vi "sort files in folder by integer in filename.vi"(11 "subarray":string[](array[string])) -> (3 "elements":string[](array[string]))   [LabVIEW 2020]
uses:
  <userlib>/_OpenG.lib/array/array.llb/Sort 1D Array (I32)__ogtk.vi
  <userlib>/_OpenG.lib/array/array.llb/Index 1D Array Elements (String)__ogtk.vi
panel:
  out "number":i32
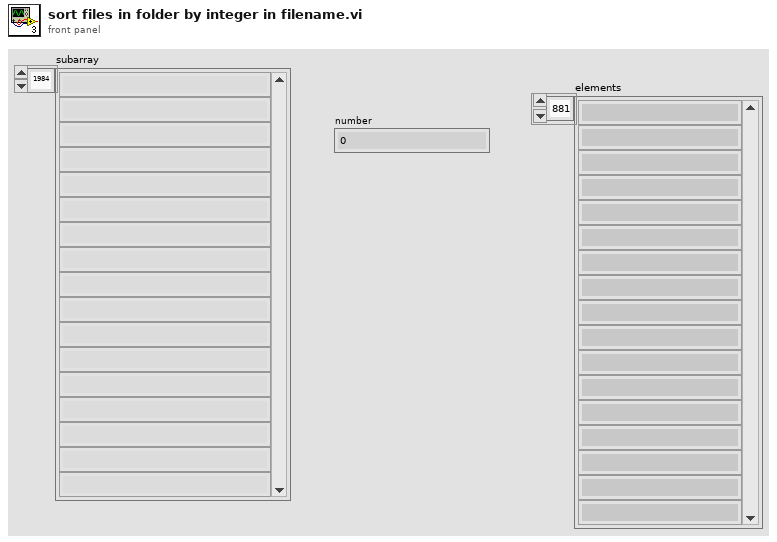
[diagram p1: front panel]
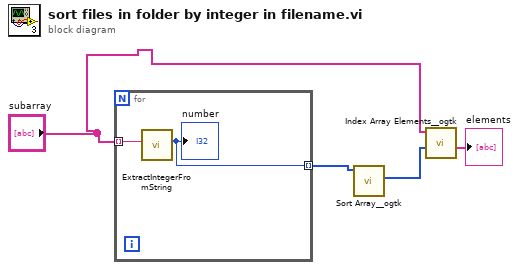
[diagram p0: block diagram]
diagram:
  n1 = for {
    tunnel: "subarray" -> [w6] mode=indexing
    tunnel: [w5] -> w4 mode=indexing
    n2 = call "ExtractIntegerFromString.vi"("String"=w6) -> ("number"=w5:i32)  [unwired: 10 in]
    "number" <- w5
  }
  n3 = call-poly <userlib>:"Sort Array__ogtk.vi"("Array in"=w4) -> ("Sorted Pointers"=w2:i32[])  [unwired: 9 in, 1 out]
  n4 = call-poly <userlib>:"Index Array Elements__ogtk.vi"("indices"=w2, "array"="subarray") -> ("elements"=→"elements":string[])  [unwired: 9 in]
